vi "ControlActivateSolenoidsGlobal (1).vi"() -> ()   [LabVIEW 2017]
panel:
  out "ActivateSolenoids":bool
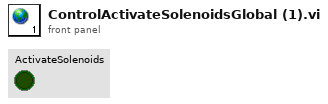
[diagram p1: front panel]
diagram:
